vi "req_headers.vi"(11 "Input":T1) -> (0 "Output":T1, 3 "JSON string":string)   [LabVIEW 2019]
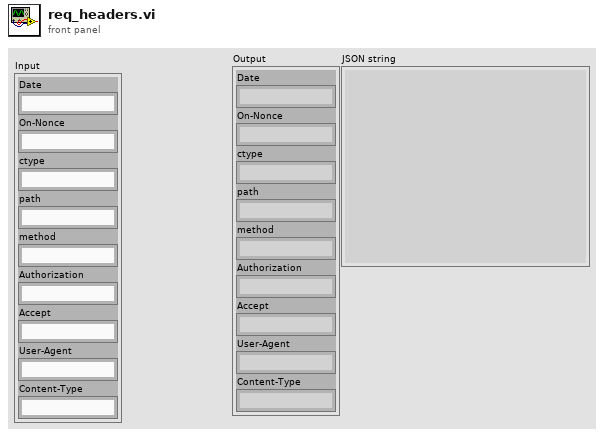
[diagram p1: front panel]
types:
  T1 = cluster{"Date":string, "On-Nonce":string, "ctype":string, "path":string, "method":string, "Authorization":string, "Accept":string, "User-Agent":string, "Content-Type":string}
  T2 = cluster{"Content-Type":string, "Date":string, "On-Nonce":string, "Authorization":string, "User-Agent":string, "Accept":string}
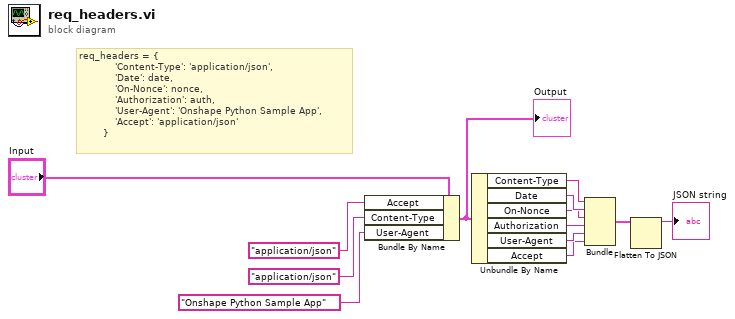
[diagram p0: block diagram]
diagram:
  # "req_headers = {\n            'Content-Type': 'application/json',\n            'Date': date,\n            'On-Nonce': nonce,\n            'Authorization': auth,\n            'User-Agent': 'Onshape Python Sample App',\n            'Accept': 'application/json'\n        }"
  n1 = Bundle By Name(cluster="Input", "Accept"="application/json" ("Content-Type"), "Content-Type"="application/json" ("Accept"), "User-Agent"="Onshape Python Sample App") -> (w9:T1)
  "Output" <- w9
  n2 = Unbundle By Name(w9) -> ("Content-Type"=w7:string, "Date"=w6:string, "On-Nonce"=w5:string, "Authorization"=w4:string, "User-Agent"=w3:string, "Accept"=w2:string)
  n3 = Bundle("Content-Type"=w7, "Date"=w6, "On-Nonce"=w5, "Authorization"=w4, "User-Agent"=w3, "Accept"=w2) -> (w1:T2)  [unwired: 1 in]
  n4 = Flatten To JSON(anything=w1) -> (JSON string=→"JSON string":string)  [unwired: 2 in, 1 out]
